vi "admin_settings.vi"() -> ()   [LabVIEW 2017]
panel:
  out "pass":string
  out "user":string
  out "Testing Mode":bool
  out "NI 2":i64
  out "NI 1":i64
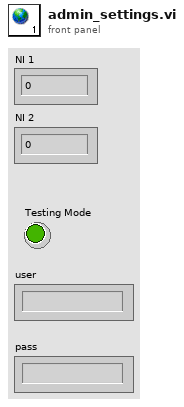
[diagram p1: front panel]
diagram:
